vi "RemoveQuotes.vi"(10 "replace string (\"\")":string="'", 11 "Input String in":string) -> (3 "Input String out":string)   [LabVIEW 2014, in "TableLogger_Actor.lvlib" / "TableLogger_Actor.lvclass"]
uses:
  TableLogger_Actor.lvclass
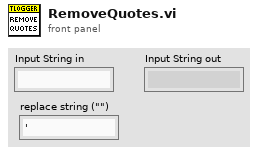
[diagram p1: front panel]
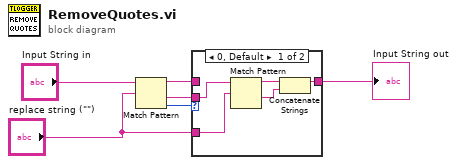
[diagram p0: block diagram]
diagram:
  n1 = Match Pattern(string="Input String in", regular expression="replace string (\"\")") -> (before substring=w2:string, after substring=w3:string, offset past match=w1:i32)  [unwired: 2 out]
  n2 = case shown="0, Default" w1 {
    tunnel: "replace string (\"\")" -> [w9 _]
    tunnel: w2 -> [_ w12]
    tunnel: [w8 w12] -> w5
    tunnel: w3 -> [w11 _]
    frame 0, Default {
      n3 = Match Pattern(string=w11, regular expression=w9) -> (before substring=w10:string, after substring=w7:string)  [unwired: 3 out]
      n4 = Concatenate Strings(w10, w7) -> (w8:string)
    }
    frame -1 {
    }
  }
  "Input String out" <- w5
